vi "File System Paths_FS-Scope SP.vi"(8 "error in":errorcluster) -> (0 "error out":errorcluster, 2 "DynamicVIs":T1, 3 "FilePaths":T2)   [LabVIEW 2012]
doc: "功能性全局。\n存储文件路径和动态VI路径。\n文件：\nChannels.bin\nTasks.bin\nDevices.bin\nSystemConstant.ini\n动态VI:\nRead Data-TCP\nWrite Command-TCP"
uses:
  System Paths_FS-Scope SP.ctl
  Dynamic VI Paths_FS-Scope SP.ctl
panel:
  in  "InitDynamicVIs":T1
  in  "InitPaths":T2
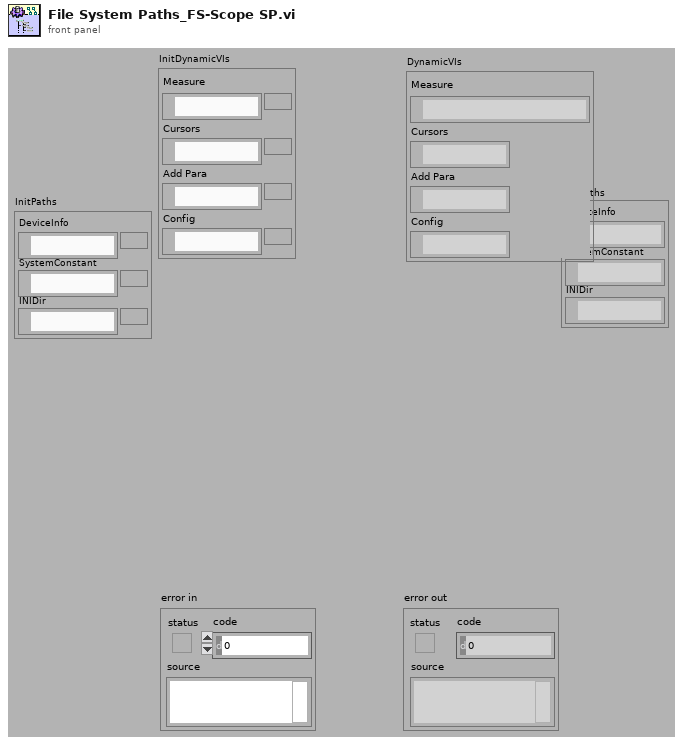
[diagram p1: front panel]
types:
  T1 = typedef "Dynamic VI Paths_FS-Scope SP.ctl" = cluster{"Measure":path, "Cursors":path, "Add Para":path, "Config":path}
  T2 = typedef "System Paths_FS-Scope SP.ctl" = cluster{"DeviceInfo":path, "SystemConstant":path, "INIDir":path}
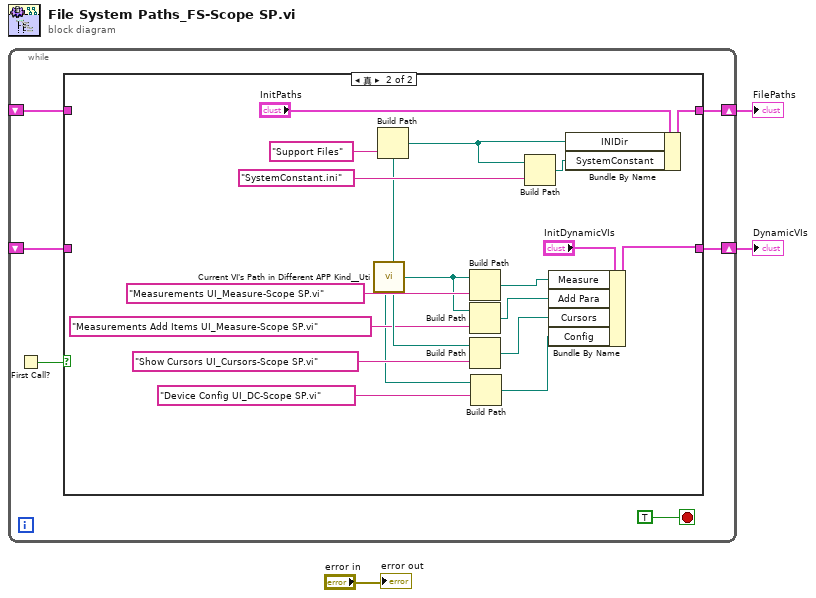
[diagram p0: block diagram]
diagram:
  n1 = while {
    shift-right: [w7] -> w3
    shift-left: _ -> [w6]
    shift-right: [w4] -> w2
    shift-left: _ -> [w5]
    stop <- TRUE stop-if-true
    n2 = First Call?() -> (First Call?: T/F=w9:bool)
    n3 = case shown="真" w9 {
      tunnel: [w11 w30] -> w7
      tunnel: w6 -> [w11 _]
      tunnel: w5 -> [w10 _]
      tunnel: [w10 w28] -> w4
      frame False {
      }
      frame True {
        n4 = call "Current VI's Path in Different APP Kind__Uti.vi"() -> ("Config"=w13:path, "Files"=w18:path, "Measure"=w16:path, "Cursor"=w19:path)  [unwired: 6 out]
        n5 = Build Path(base path=w18, name or relative path="Support Files") -> (appended path=w20:path)
        n6 = Build Path(base path=w16, name or relative path="Measurements UI_Measure-Scope SP.vi") -> (appended path=w26:path)
        n7 = Build Path(base path=w16, name or relative path="Measurements Add Items UI_Measure-Scope SP.vi") -> (appended path=w17:path)
        n8 = Build Path(base path=w19, name or relative path="Show Cursors UI_Cursors-Scope SP.vi") -> (appended path=w24:path)
        n9 = Build Path(base path=w13, name or relative path="Device Config UI_DC-Scope SP.vi") -> (appended path=w12:path)
        n10 = Build Path(base path=w20, name or relative path="SystemConstant.ini") -> (appended path=w21:path)
        n11 = Bundle By Name(cluster="InitDynamicVIs", "Measure"=w26, "Add Para"=w17, "Cursors"=w24, "Config"=w12) -> (w28:T1)
        n12 = Bundle By Name(cluster="InitPaths", "INIDir"=w20, "SystemConstant"=w21) -> (w30:T2)
      }
    }
  }
  "FilePaths" <- w3
  "DynamicVIs" <- w2
  "error out" <- "error in"
